vi "Pyramid_path.vi"() -> ()   [LabVIEW 2015]
uses:
  <vilib>/Math Plots/3D Math Plots/3D Scatter/3D Scatter XCtrl/3D Scatter.xctl
  <vilib>/Math Plots/3D Math Plots/3D Comet/3D Comet XCtrl/3D Comet.xctl
  Globals.vi
panel:
  in  "Tab Control":enum32{"Reference ", "Page 2"}(tab)
  in  "Ring":u16(ring) items=["Pyramid", "NX Pattern"]
  in  "Save Button":bool
  out "Calculated Depth":dbl
  in  "vangle":dbl
  in  "overlap":dbl
  in  "increment":dbl
  in  "width":dbl
  in  "layers":dbl
  in  "height":dbl
  in  "stop":bool
  in  "Min_dist":dbl
  out "3D Scatter 2":refnum<class "3D Plot Datatype.lvclass">[](xcontrol)
  out "3D Comet":refnum<class "3D Plot Datatype.lvclass">[](xcontrol)
  in  "refresh":bool
  in  "interpolate":bool
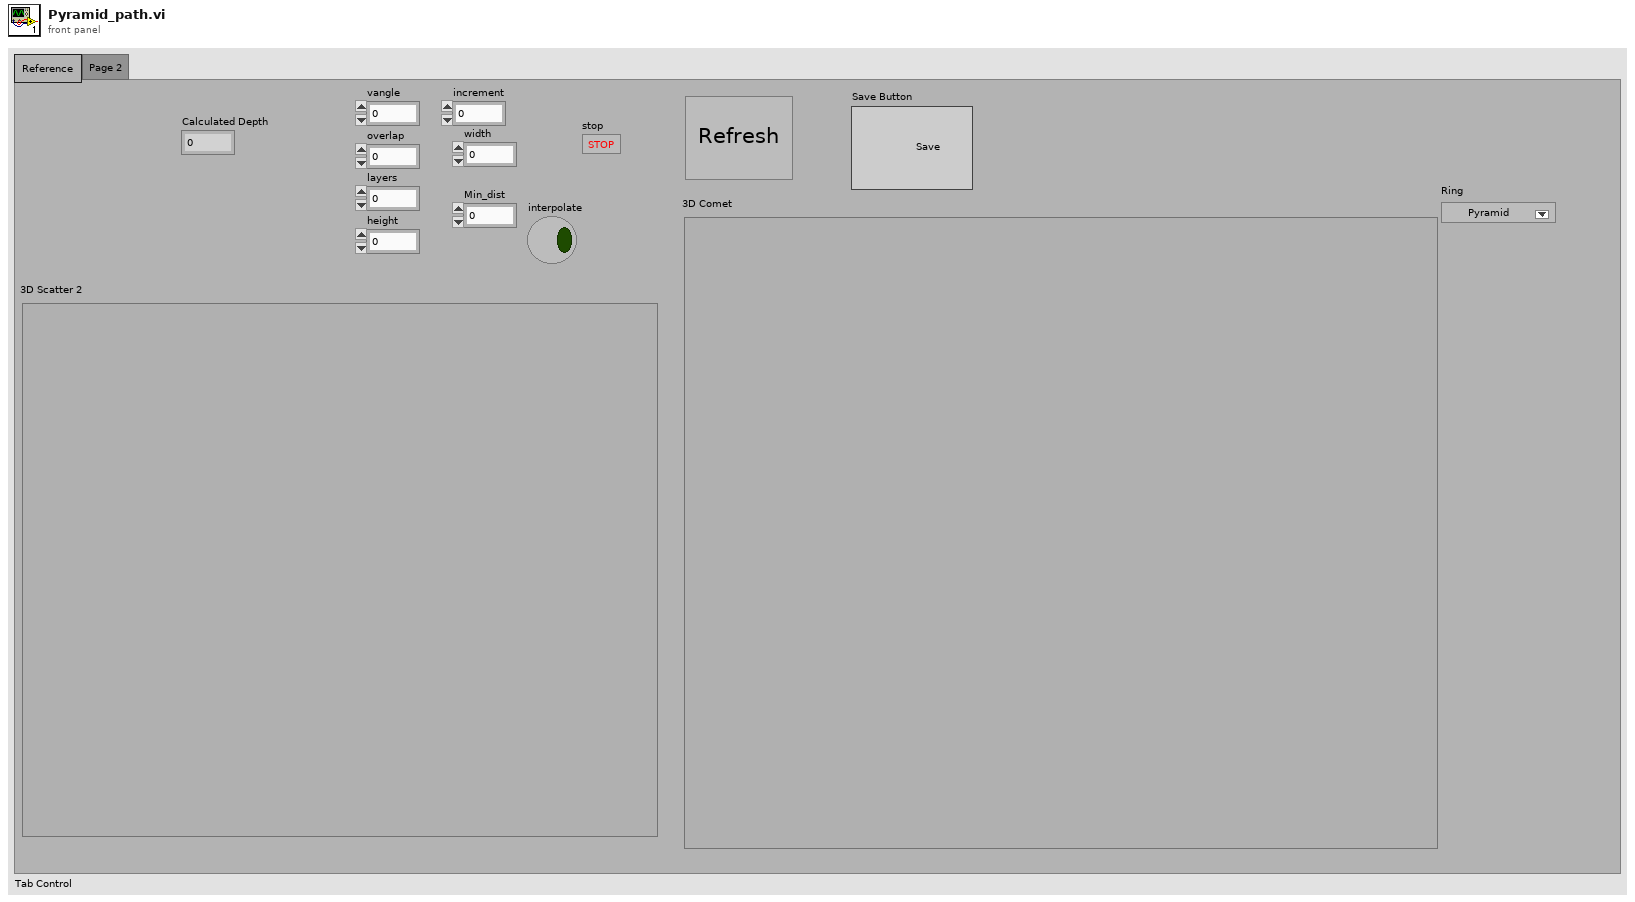
[diagram p1: front panel]
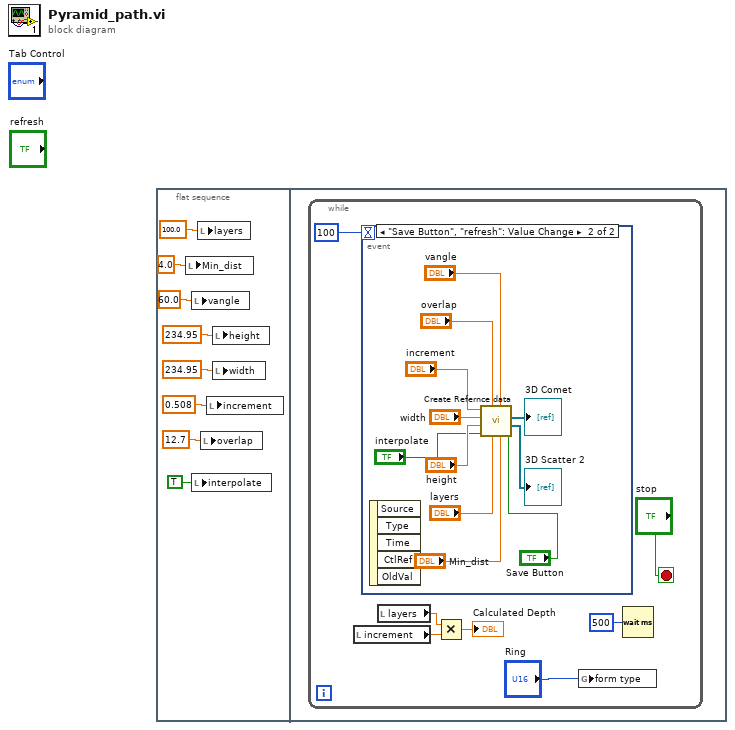
[diagram p0: block diagram]
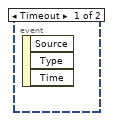
[diagram p2: hidden frame]
diagram:
  n1 = flat-sequence {
    frame #0 {
      n2 = local write "Min_dist"(4.0 ("vangle")) -> ()
      n3 = local write "vangle"(60.0 ("vangle")) -> ()
      n4 = local write "interpolate"(TRUE ("Interpolate")) -> ()
      n5 = local write "layers"(100.0 ("vangle")) -> ()
      n6 = local write "overlap"(12.7 ("vangle")) -> ()
      n7 = local write "increment"(0.508 ("vangle")) -> ()
      n8 = local write "height"(234.95 ("vangle")) -> ()
      n9 = local write "width"(234.95 ("vangle")) -> ()
    }
    frame #1 {
      n10 = while {
        stop <- "stop" stop-if-true
        n11 = local read "increment"() -> (w10:dbl)
        n12 = event shown="[1] \"Save Button\", \"refresh\": Value Change" {
          selector: _ -> [_ _]
          dyn-events: _ -> [_ _]
          timeout: 100 -> [_ _]
          event Timeout {
            n13 = event-data() -> ()  [unwired: 1 in, 3 out]
          }
          event "Save Button", "refresh": Value Change {
            n14 = event-data() -> ()  [unwired: 1 in, 5 out]
            n15 = call "Create Refernce data.vi"("Save Button"="Save Button", "Min_dist"="Min_dist", "vangle"="vangle", "layers"="layers", "overlap"="overlap", "Interpolate"="interpolate", "height"="height", "width"="width", "increment"="increment") -> ("Reference"=→"3D Scatter 2":refnum<class "3D Plot Datatype.lvclass">[], "3D Comet"=→"3D Comet":refnum<class "3D Plot Datatype.lvclass">[])  [unwired: 1 in]
          }
        }
        n16 = local read "layers"() -> (w11:dbl)
        n17 = Multiply(x=w11, y=w10) -> (x*y=→"Calculated Depth":dbl)
        n18 = global write "Globals.vi" "form type"("Ring") -> ()
        n19 = Wait (ms)(milliseconds to wait=u32 500) -> ()  [unwired: 1 out]
      }
    }
  }
